vi "Agilent 4263X Single Measurement.vi"() -> ()   [LabVIEW 2016]
doc: "This Example VI configures the instrument to take one measurement of the specified functions.\n\nThe bus trigger (:TRIG) is used to trigger the measurements which is then read back to the computer.\n\nThe instrument should be first initialized with the Initialize VI (ID query and Reset should be set to yes).\n\nThis VI sets the primary and secondary measurement types along with the trigger mode (bus) and averaging rate. The VI then reads the primary and secondary measurments."
uses:
  <instrlib>/Agilent 4263X/Agilent 4263X.lvlib
panel:
  in  "VISA resource name":refnum<visa-resource-name>
  in  "averaging count (1)":i16=1 min=1 max=256 step=1
  out "secondary reading":dbl format="%.5e"
  out "primary reading":dbl format="%.5e"
  out "status":u16
  in  "function (Z - Angle:0)":u16(ring) items=["Z - Angle", "R - X", "Y - Angle", "G - B", "CP - D", "CP - Q", "CP - G", "CS - D", "CS - Q", "CS - RS", "LP - D", "LP - Q", "LP - G", "LS - D", "LS - Q", "LS - RS", "LS - DCR (option 001 only)", "LP - DCR (option 001 only)", "L2 - N (option 001 only)", "L2 - M (option 001 only)", "L2 - R2 (option 001 only)"]
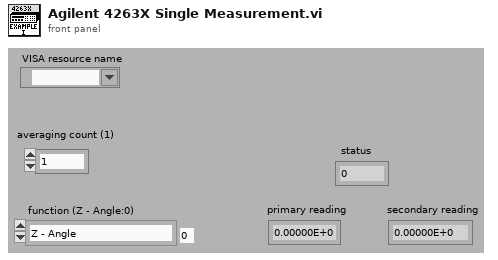
[diagram p1: front panel]
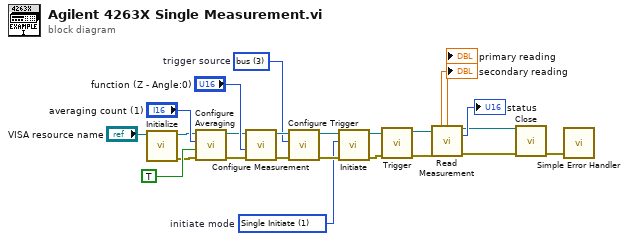
[diagram p0: block diagram]
diagram:
  w1 = u16 3 items=["internal", "external", "manual", "bus"]  # trigger source
  w4 = u16 1 items=["Continuous Initiate", "Single Initiate", "Stop Continuous"]  # initiate mode
  n1 = call <instrlib>:"Initialize.vi"("VISA resource name"="VISA resource name") -> ("error out"=w10:errorcluster, "VISA resource name out"=w9:refnum<visa-resource-name>)  [unwired: 9 in]
  n2 = call <instrlib>:"Configure Averaging.vi"("error in (no error)"=w10, "Enable Averge Mode  (on:T)"=TRUE, "Average count (1)"="averaging count (1)", "VISA resource name"=w9) -> ("error out"=w14:errorcluster, "VISA resource name out"=w13:refnum<visa-resource-name>)  [unwired: 6 in]
  n3 = call <instrlib>:"Configure Measurement.vi"("error in (no error)"=w14, "function (Z - Angle:0)"="function (Z - Angle:0)", "VISA resource name"=w13) -> ("error out"=w21:errorcluster, "VISA resource name out"=w2:refnum<visa-resource-name>)  [unwired: 7 in]
  n4 = call <instrlib>:"Configure Trigger.vi"("error in (no error)"=w21, "trigger source (int:0)"=w1, "VISA resource name"=w2) -> ("error out"=w18:errorcluster, "VISA resource name out"=w17:refnum<visa-resource-name>)  [unwired: 7 in]
  n5 = call <instrlib>:"Initiate.vi"("error in (no error)"=w18, "initiate mode (0:continuous)"=w4, "VISA resource name"=w17) -> ("error out"=w15:errorcluster, "VISA resource name out"=w16:refnum<visa-resource-name>)  [unwired: 7 in]
  n6 = call <instrlib>:"Trigger.vi"("error in (no error)"=w15, "VISA resource name"=w16) -> ("error out"=w20:errorcluster, "VISA resource name out"=w19:refnum<visa-resource-name>)  [unwired: 8 in]
  n7 = call <instrlib>:"Read Measurement.vi"("VISA resource name"=w19, "error in (no error)"=w20) -> ("VISA resource name out"=w6:refnum<visa-resource-name>, "status"=→"status":u16, "primary reading"=→"primary reading":dbl, "secondary reading"=→"secondary reading":dbl, "error out"=w5:errorcluster)  [unwired: 7 in, 2 out]
  n8 = call <instrlib>:"Close.vi"("error in (no error)"=w5, "VISA resource name"=w6) -> ("error out"=w3:errorcluster)  [unwired: 9 in]
  n9 = call <vilib>:"Simple Error Handler.vi"("error in (no error)"=w3) -> ()  [unwired: 4 in, 5 out]
